vi "IdentityCheck.vi"(8 "error in (no error)":errorcluster, 11 "Tektronix RSA5106A in":refnum<class "Tektronix RSA5106A.lvclass">) -> (0 "error out":errorcluster, 3 "Tektronix RSA5106A out":refnum<class "Tektronix RSA5106A.lvclass">)   [LabVIEW 2013, in "Tektronix RSA5106A.lvclass"]
uses:
  Tektronix RSA5106A.lvclass
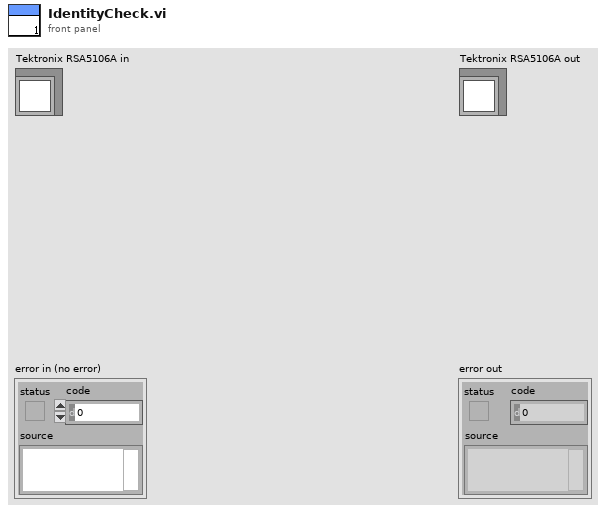
[diagram p1: front panel]
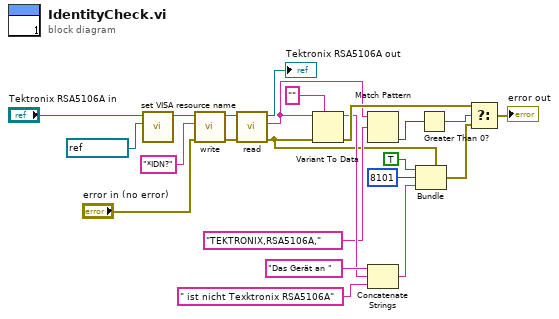
[diagram p0: block diagram]
diagram:
  n1 = call-dynamic "set VISA resource name.vi"("VISA resource name"=refnum<visa-resource-name> "COM4", "DeviceInterface (Eingang)"="Tektronix RSA5106A in") -> ("DeviceInterface (Ausgang)"=w1:refnum<class "Tektronix RSA5106A.lvclass">)  [unwired: 8 in, 1 out]
  n2 = call-dynamic "write.vi"("error in (no error)"="error in (no error)", "String to send"="*IDN?" ("Reset Command"), "Tektronix RSA5106A in"=w1) -> ("error out"=w8:errorcluster, "Tektronix RSA5106A out"=w7:refnum<class "Tektronix RSA5106A.lvclass">)  [unwired: 7 in]
  n3 = call-dynamic "read.vi"("error in (no error)"=w8, "Tektronix RSA5106A in"=w7) -> ("error out"=w4:errorcluster, "Return String"=w5:string, "Tektronix RSA5106A out"=→"Tektronix RSA5106A out":refnum<class "Tektronix RSA5106A.lvclass">)  [unwired: 7 in]
  n4 = Variant To Data(error in=w4, type="" ("input"), Variant=w5) -> (data=w12:string, error out=w18:errorcluster)
  n5 = Match Pattern(string=w5, regular expression="TEKTRONIX,RSA5106A,") -> (offset past match=w21:i32)  [unwired: 1 in, 3 out]
  n6 = Concatenate Strings("Das Gerät an " ("string"), w12, " ist nicht Texktronix RSA5106A" ("string")) -> (w15:string)
  n7 = Bundle(cluster=w4, "status"=TRUE, "code"=8101, "source"=w15) -> (w16:errorcluster)
  n8 = Greater Than 0?(x=w21) -> (x > 0?=w20:bool)
  n9 = Select(t=w18, s=w20, f=w16) -> (s? t:f=→"error out":errorcluster)
